vi "RC_Test.vi"() -> ()   [LabVIEW 2013]
uses:
  Data/TypeDefs/DynamixelCycleTracker.ctl
  Data/TypeDefs/Rudder Set Suggestions.ctl
  Data/TypeDefs/HindbrainControlOptions.ctl
  Data/TypeDefs/MotorSetup.ctl
  Data/TypeDefs/DynamixelSetupInfo.ctl
  <vilib>/FPGAPlugInAG/myRIO-1900/niLvFpga_Open_myRIO-1900.vi
  <vilib>/rvi/interface/common/dynamic/niFpgaDynamicAddResources.vi
  <vilib>/rvi/interface/nirviOpenFPGA/nirviOpenFPGA.xnode
  FPGA Bitfiles/AutonomousSailbo_FPGATarget_myRIOPWMDecoder_0snwDOwOU4s.lvbitx
  FPGA_Code/myRIO_PWM_Decoder.vi
  <instrlib>/Dynamixel Motor/Dynamixel Motor.lvlib
panel:
  out "Position Sail 2":dbl
  out "Position Sail 1":dbl
  out "Calibration loop counter":i32
  in  "Sail 2 Bound Offset":dbl=800.0
  in  "Sail 1 Bound Offset":dbl=800.0
  in  "Dynamixel Bounds":T1={"Main Dynamixel Set Data"={"Lower Winch Bound (deg)"=0.0, "Upper Winch Bound (deg)"=0.0}, "Rudder Dynamixel Set Data"={"Lower Winch Bound (deg)"=15.0, "Upper Winch Bound (deg)"=60.0}, "Jib Dynamixel Set Data"={"Lower Winch Bound (deg)"=0.0, "Upper Winch Bound (deg)"=0.0}}
  in  "Sail 1 Lower Bound":dbl
  in  "Sail 2 Lower Bound":dbl
  in  "Stop Calibration":bool
  in  "Mode control":T3=enum."RC_control"
  out "Motors IDs Found":u8[](array[numeric])
  out "Commanded rudder value":T4 min=-0.95 max=0.95 scale=1.0..-1.0
  out "Commanded sail value":dbl
  out "Write loop counter":i32
  out "Updated Dynamixle Cycles":T5
  out "Dynamixel Positions (deg)":dbl[](array[numeric])
  out "Read loop counter":i32
  in  "Stop reading":bool
  in  "Stop writing":bool
  in  "VISA resource name":refnum<visa-resource-name>="ASRL3::INSTR"
  # "Read from RC Controller"
  # "Read from Dynamixels"
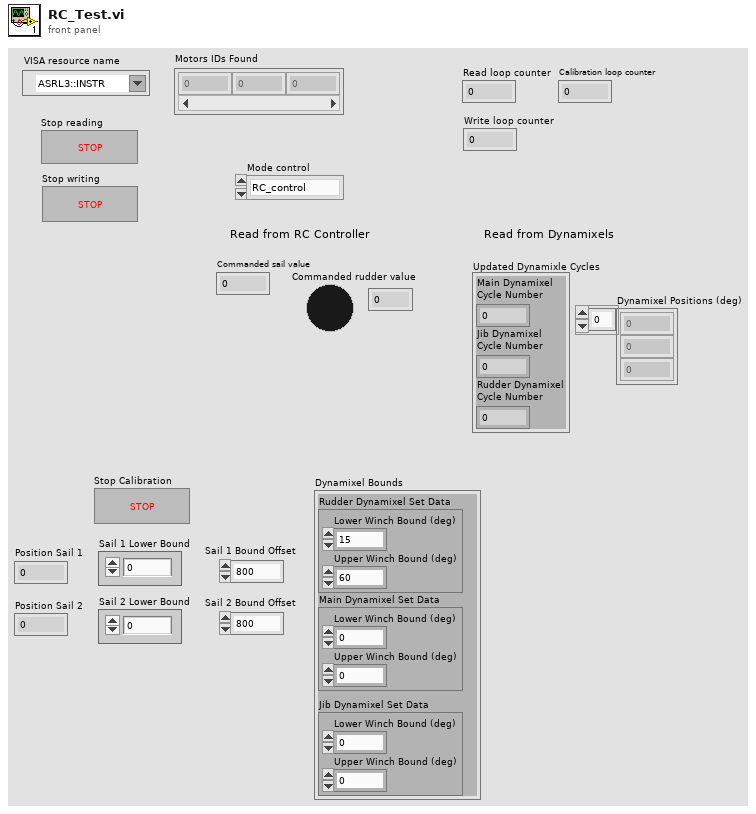
[diagram p1: front panel]
types:
  T1 = typedef "MotorSetup.ctl" = cluster{"Main Dynamixel Set Data":T2, "Rudder Dynamixel Set Data":T2, "Jib Dynamixel Set Data":T2}
  T2 = typedef "DynamixelSetupInfo.ctl" = cluster{"Lower Winch Bound (deg)":dbl, "Upper Winch Bound (deg)":dbl}
  T3 = typedef "HindbrainControlOptions.ctl" = enum16{"code_control", "RC_control", "hand_control"}
  T4 = typedef "Rudder Set Suggestions.ctl" = dbl
  T5 = typedef "DynamixelCycleTracker.ctl" = cluster{"Main Dynamixel\nCycle Number":i32, "Jib Dynamixel\nCycle Number":i32, "Rudder Dynamixel\nCycle Number":i32}
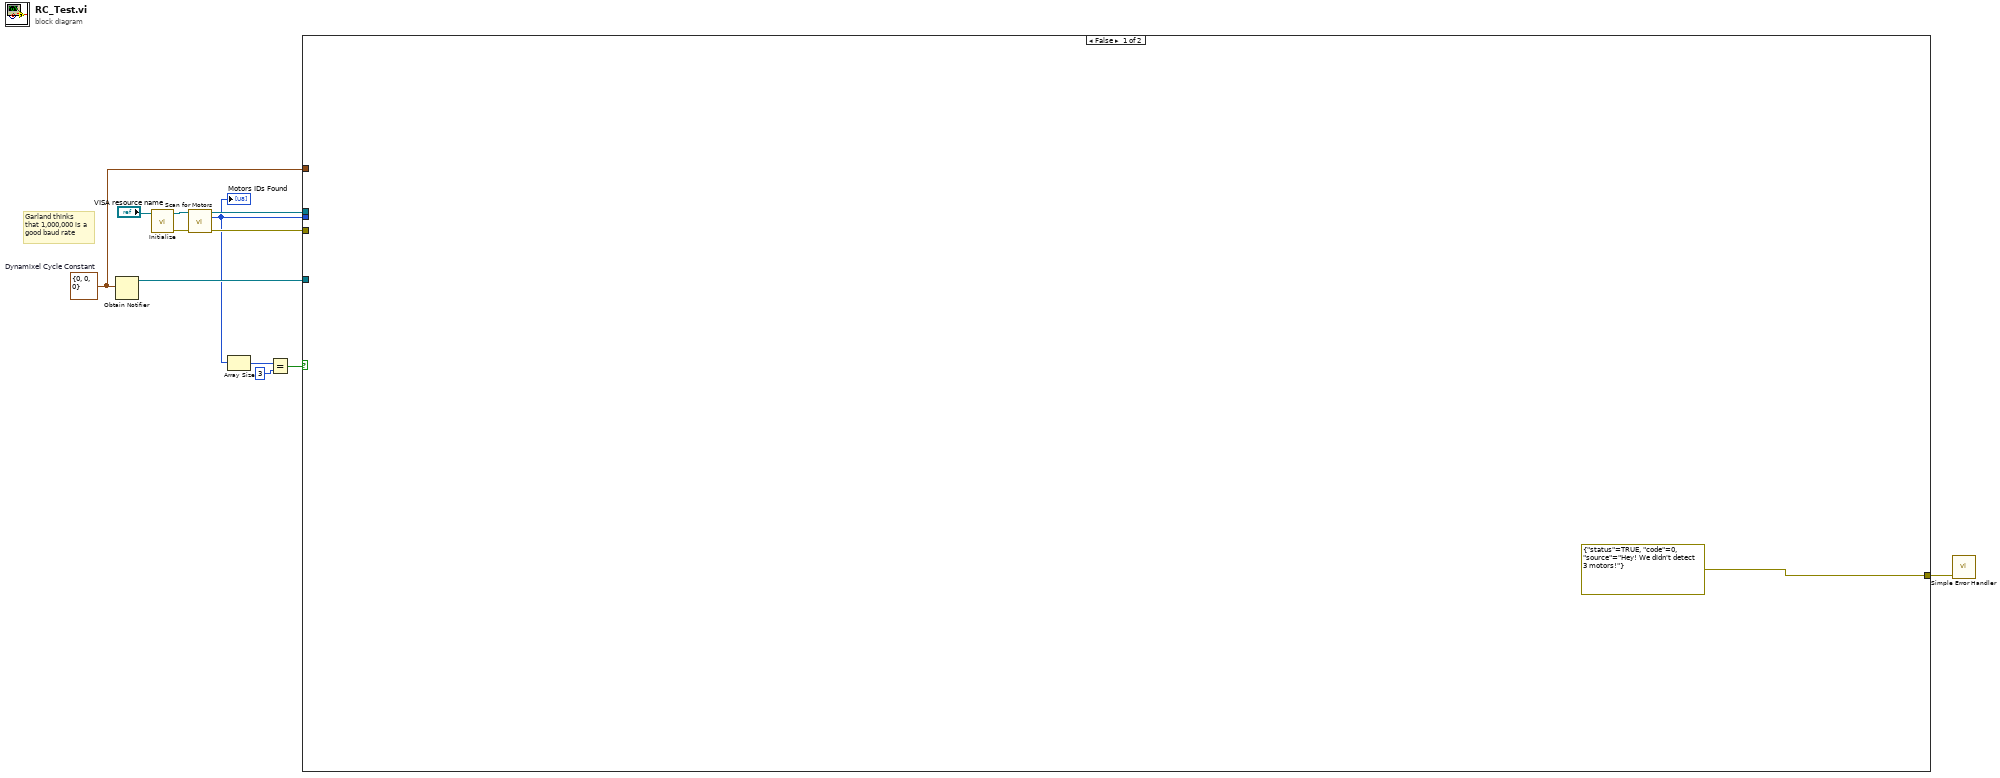
[diagram p0: block diagram]
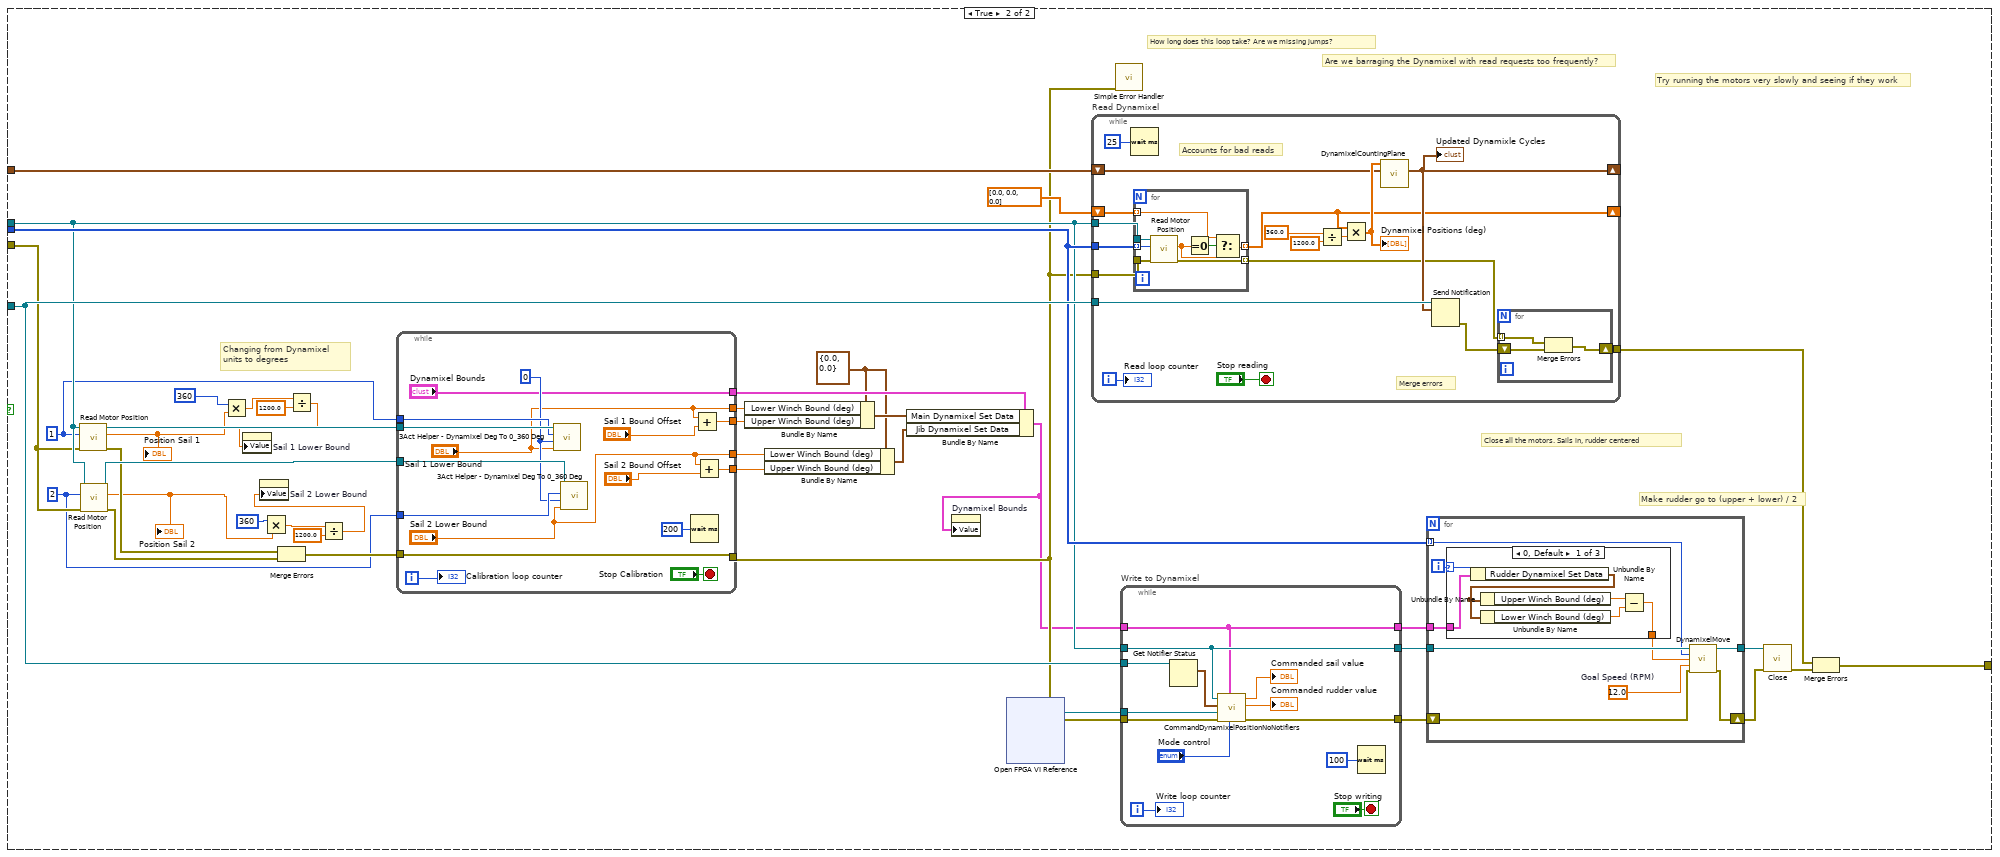
[diagram p2: hidden frame]
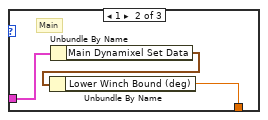
[diagram p3: hidden frame]
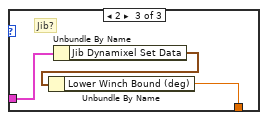
[diagram p4: hidden frame]
diagram:
  w8 = T5 {"Main Dynamixel\nCycle Number"=0, "Jib Dynamixel\nCycle Number"=0, "Rudder Dynamixel\nCycle Number"=0}  # Dynamixel Cycle Constant
  # "Garland thinks that 1,000,000 is a good baud rate"
  n1 = Obtain Notifier(notification data type=w8) -> (notifier out=w12:refnum<notifier>)  [unwired: 3 in, 2 out]
  n2 = call <instrlib>:"Initialize.vi"("VISA resource name"="VISA resource name") -> ("error out"=w10:errorcluster, "VISA resource name out"=w9:refnum<visa-resource-name>)  [unwired: 9 in]
  n3 = call <instrlib>:"Scan for Motors.vi"("VISA resource name"=w9, "error in (no error)"=w10) -> ("VISA resource name out"=w7:refnum<visa-resource-name>, "Motors IDs Found"=w1:u8[], "error out"=w6:errorcluster)  [unwired: 11 in]
  "Motors IDs Found" <- w1
  n4 = Array Size(array=w1) -> (size(s)=w5:i32)
  n5 = Equal?(x=w5, y=3) -> (x = y?=w4:bool)
  n6 = case shown="False" w4 {
    tunnel: w12 -> [_ w54]
    tunnel: w8 -> [_ w53]
    tunnel: w1 -> [_ w51]
    tunnel: w7 -> [_ w43]
    tunnel: w6 -> [_ w40]
    tunnel: [errorcluster {"status"=TRUE, "code"=0, "source"="Hey! We didn't detect 3 motors!"} ("error IO") w27] -> w2
    frame False {
    }
    frame True {
      w28 = u8 2 ("Motor ID (0)")
      w29 = u8 1 ("Motor ID (0)")
      w36 = T2 {"Lower Winch Bound (deg)"=0.0, "Upper Winch Bound (deg)"=0.0} ("Main Dynamixel Set Data")
      # "Changing from Dynamixel units to degrees"
      # "Make rudder go to (upper + lower) / 2"
      # "Close all the motors. Sails in, rudder centered"
      # "Try running the motors very slowly and seeing if they work"
      # "Are we barraging the Dynamixel with read requests too frequently?"
      # "How long does this loop take? Are we missing jumps?"
      n7 = call <instrlib>:"Read Motor Position.vi"("error in (no error)"=w40, "Motor ID (0)"=w29, "VISA resource name"=w43) -> ("error out"=w24:errorcluster, "Position (deg)"=w19:dbl, "VISA resource name out"=w42:refnum<visa-resource-name>)  [unwired: 6 in]
      "Position Sail 1" <- w19
      n8 = call <instrlib>:"Read Motor Position.vi"("error in (no error)"=w40, "Motor ID (0)"=w28, "VISA resource name"=w43) -> ("error out"=w25:errorcluster, "Position (deg)"=w21:dbl, "VISA resource name out"=w41:refnum<visa-resource-name>)  [unwired: 6 in]
      "Position Sail 2" <- w21
      n9 = Multiply(x=u16 360, y=w19) -> (x*y=w17:dbl)
      n10 = Multiply(x=u16 360, y=w21) -> (x*y=w15:dbl)
      n11 = Merge Errors(w24, w25) -> (w31:errorcluster)
      n12 = Divide(x=w17, y=1200.0) -> (x/y=w18:dbl)
      n13 = property on="Sail 1 Lower Bound" class="DigNum (strict)"("Value"=w18) -> ()  [unwired: 2 in, 2 out]
      n14 = Divide(x=w15, y=1200.0) -> (x/y=w20:dbl)
      n15 = property on="Sail 2 Lower Bound" class="DigNum (strict)"("Value"=w20) -> ()  [unwired: 2 in, 2 out]
      n16 = while {
        tunnel: w42 -> [w71]
        tunnel: w41 -> [w70]
        tunnel: w29 -> [w69]
        tunnel: w28 -> [w68]
        tunnel: ["Dynamixel Bounds"] -> w39
        tunnel: ["Sail 1 Lower Bound"] -> w35
        tunnel: ["Sail 2 Lower Bound"] -> w34
        tunnel: [w63] -> w33
        tunnel: [w62] -> w32
        tunnel: w31 -> [w59]
        tunnel: [w59] -> w30
        i -> [w58]
        stop <- "Stop Calibration" stop-if-true
        w67 = 0 ("Dynamixel Cycle Number")
        n17 = call "3Act Helper - Dynamixel Deg To 0_360 Deg.vi"("Dynamixel Setpoint In (deg)"="Sail 1 Lower Bound", "Dynamixel Cycle Number"=w67, "Motor ID"=w69, "VISA resource name"=w71) -> ()  [unwired: 6 in, 2 out]
        n18 = call "3Act Helper - Dynamixel Deg To 0_360 Deg.vi"("Dynamixel Setpoint In (deg)"="Sail 2 Lower Bound", "Dynamixel Cycle Number"=w67, "Motor ID"=w68, "VISA resource name"=w70) -> ()  [unwired: 6 in, 2 out]
        n19 = Wait (ms)(milliseconds to wait=u32 200) -> ()  [unwired: 1 out]
        n20 = Add(x="Sail 1 Lower Bound", y="Sail 1 Bound Offset") -> (x+y=w63:dbl)
        n21 = Add(x="Sail 2 Lower Bound", y="Sail 2 Bound Offset") -> (x+y=w62:dbl)
        "Calibration loop counter" <- w58
      }
      n22 = Bundle By Name(cluster=w36, "Lower Winch Bound (deg)"=w35, "Upper Winch Bound (deg)"=w33) -> (w38:T2)
      n23 = Bundle By Name(cluster=w36, "Lower Winch Bound (deg)"=w34, "Upper Winch Bound (deg)"=w32) -> (w37:T2)
      n24 = Bundle By Name(cluster=w39, "Main Dynamixel Set Data"=w38, "Jib Dynamixel Set Data"=w37) -> (w26:T1)
      n25 = property on="Dynamixel Bounds" class="Clust (strict)"("Value"=w26) -> ()  [unwired: 2 in, 2 out]
      n26 = xnode "Open FPGA VI Reference"() -> ("FPGA VI Reference Out"=w55:refnum<k20>)  [unwired: 2 in, 1 out]
      n27 = while "Read Dynamixel" {
        tunnel: w43 -> [w121]
        shift-right: [w119] -> _
        shift-left: w53 -> [w107]
        tunnel: w54 -> [w120]
        tunnel: w51 -> [w117]
        tunnel: w30 -> [w122]
        shift-right: [w109] -> _
        shift-left: dbl[] [0.0, 0.0, 0.0] -> [w108]
        tunnel: [w105] -> w45
        i -> [w115]
        stop <- "Stop reading" stop-if-true
        # "Accounts for bad reads"
        # "Merge errors"
        n28 = Wait (ms)(milliseconds to wait=u32 25) -> ()  [unwired: 1 out]
        n29 = for {
          tunnel: w121 -> [w133]
          tunnel: [w127] -> w109 mode=indexing
          tunnel: w117 -> [w130] mode=indexing
          tunnel: w122 -> [w132]
          tunnel: [w131] -> w116 mode=indexing
          tunnel: w108 -> [w126] mode=indexing
          n30 = call <instrlib>:"Read Motor Position.vi"("error in (no error)"=w132, "Motor ID (0)"=w130, "VISA resource name"=w133) -> ("error out"=w131:errorcluster, "Position (deg)"=w128:dbl)  [unwired: 6 in, 1 out]
          n31 = Equal To 0?(x=w128) -> (x = 0?=w129:bool)
          n32 = Select(t=w126, s=w129, f=w128) -> (s? t:f=w127:dbl)
        }
        n33 = Divide(x=360.0, y=1200.0) -> (x/y=w110:dbl)
        n34 = Multiply(x=w109, y=w110) -> (x*y=w112:dbl[])
        "Dynamixel Positions (deg)" <- w112
        n35 = call "DynamixelCountingPlane.vi"("Dynamixel Cycles"=w107, "Dynamixel Read Positions"=w112) -> ("Updated Dynamixle Cycles"=w119:T5)  [unwired: 9 in]
        "Updated Dynamixle Cycles" <- w119
        n36 = Send Notification(notification=w119, notifier=w120) -> (error out=w106:errorcluster)  [unwired: 1 in, 1 out]
        n37 = for {
          tunnel: w116 -> [w123] mode=indexing
          shift-right: [w125] -> w105
          shift-left: w106 -> [w124]
          n38 = Merge Errors(w123, w124) -> (w125:errorcluster)
        }
        "Read loop counter" <- w115
      }
      n39 = call <vilib>:"Simple Error Handler.vi"("error in (no error)"=w30) -> ()  [unwired: 4 in, 5 out]
      n40 = while "Write to Dynamixel" {
        tunnel: w55 -> [w104]
        tunnel: w43 -> [w97]
        tunnel: w54 -> [w103]
        tunnel: w30 -> [w101]
        tunnel: [w100] -> w52
        tunnel: [w97] -> w50
        tunnel: [w92] -> w44
        tunnel: w26 -> [w92]
        i -> [w96]
        stop <- "Stop writing" stop-if-true
        n41 = Get Notifier Status(notifier=w103) -> (current notification=w102:T5)  [unwired: 1 in, 4 out]
        n42 = call "CommandDynamixelPositionNoNotifiers.vi"("Mode control"="Mode control", "Dynamixel Bounds"=w92, "error in"=w101, "FPGA VI Reference In"=w104, "Dynamixel Cycles"=w102, "VISA resource name"=w97) -> ("Error out"=w100:errorcluster, "Commanded rudder value"=→"Commanded rudder value":T4, "Commanded sail value"=→"Commanded sail value":dbl)  [unwired: 3 in]
        n43 = Wait (ms)(milliseconds to wait=u32 100) -> ()  [unwired: 1 out]
        "Write loop counter" <- w96
      }
      n44 = for {
        tunnel: w50 -> [w80]
        shift-right: [w79] -> w49
        shift-left: w52 -> [w78]
        tunnel: w51 -> [w76] mode=indexing
        tunnel: [w75] -> w46
        tunnel: w44 -> [w73]
        i -> [w74]
        w77 = 12.0  # Goal Speed (RPM)
        n45 = case shown="0, Default" w74 {
          tunnel: w73 -> [w85 w87 w91]
          tunnel: [w82 w86 w89] -> w72
          frame 0, Default {
            n46 = Unbundle By Name(w85) -> ("Rudder Dynamixel Set Data"=w84:T2)
            n47 = Unbundle By Name(w84) -> ("Upper Winch Bound (deg)"=w83:dbl)
            n48 = Unbundle By Name(w84) -> ("Lower Winch Bound (deg)"=w81:dbl)
            n49 = Subtract(x=w83, y=w81) -> (x-y=w82:dbl)
          }
          frame 1 {
            # "Main"
            n50 = Unbundle By Name(w87) -> ("Main Dynamixel Set Data"=w88:T2)
            n51 = Unbundle By Name(w88) -> ("Lower Winch Bound (deg)"=w86:dbl)
          }
          frame 2 {
            # "Jib?"
            n52 = Unbundle By Name(w91) -> ("Jib Dynamixel Set Data"=w90:T2)
            n53 = Unbundle By Name(w90) -> ("Lower Winch Bound (deg)"=w89:dbl)
          }
        }
        n54 = call "DynamixelMove.vi"("VISA resource name"=w80, "Motor ID (0)"=w76, "Goal Position (150 deg)"=w72, "Goal Speed (RPM)"=w77, "error in (no error)"=w78) -> ("VISA resource name out"=w75:refnum<visa-resource-name>, "error out"=w79:errorcluster)  [unwired: 9 in]
      }
      n55 = call <instrlib>:"Close.vi"("error in (no error)"=w49, "VISA resource name"=w46) -> ("error out"=w48:errorcluster)  [unwired: 9 in]
      n56 = Merge Errors(w45, w48) -> (w27:errorcluster)
    }
  }
  n57 = call <vilib>:"Simple Error Handler.vi"("error in (no error)"=w2) -> ()  [unwired: 4 in, 5 out]
